vi "Init File.vi"(8 "error in (no error)":errorcluster, 11 "[C] User Management in":refnum<class "[C] User Management.lvclass">) -> (0 "error out":errorcluster, 3 "[C] User Management out":refnum<class "[C] User Management.lvclass">)   [LabVIEW 2020, in "[C] User Management.lvlib" / "[C] User Management.lvclass"]
uses:
  [C] User Management.lvclass
  [C] User Management.lvclass/[C] User Management.ctl
  [Data] Userinfo/[Data] Userinfo Binary/[Data] Userinfo Binary.lvclass
  D:/03 GitHub/LabVIEW-User-Management/[Data] Userinfo/[Data] Abstruct Userinfo/[Data] Abstruct Userinfo.lvclass
  [Data] Recent User/[Data] Recent User.lvclass
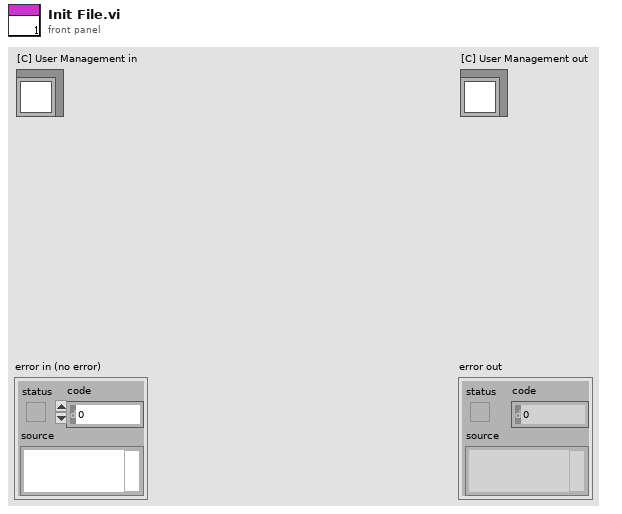
[diagram p1: front panel]
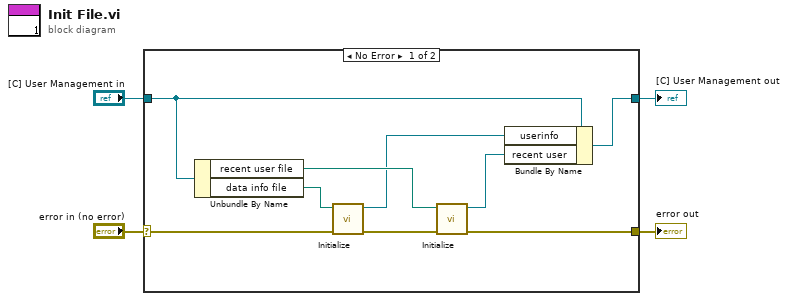
[diagram p0: block diagram]
diagram:
  n1 = case shown="No Error" "error in (no error)" {
    selector: "error in (no error)" -> [w13 w15]
    tunnel: [w9 w15] -> w3
    tunnel: [w5 w14] -> w1
    tunnel: "[C] User Management in" -> [w8 w14]
    frame No Error {
      n2 = Unbundle By Name(w8) -> ("recent user file"=w10:path, "data info file"=w12:path)
      n3 = call "Initialize.vi"("error in (no error)"=w13, "userinfo file"=w12) -> ("error out"=w11:errorcluster, "[Data] Userinfo Binary out"=w7:refnum<class "[Data] Userinfo Binary.lvclass">)  [unwired: 8 in]
      n4 = call "Initialize.vi"("error in (no error)"=w11, "recent user file"=w10) -> ("error out"=w9:errorcluster, "[Data] Recent User out"=w6:refnum<class "[Data] Recent User.lvclass">)  [unwired: 8 in]
      n5 = Bundle By Name(cluster=w8, "userinfo"=w7, "recent user"=w6) -> (w5:refnum<class "[C] User Management.lvclass">)
    }
    frame Error {
    }
  }
  "error out" <- w3
  "[C] User Management out" <- w1
